vi "niRFUtil MT Resample.vi"(0 "Waveform In":T1={"x0"=0.0, "dx"=1.0, "y"=[]} caption="input complex waveform" {"y" format="%.2f"; "dx" format="%^.2e"; "x0" format="%^.2e"}, 1 "initial sample offset (sec)":dbl format="%.2f", 7 "desired sample rate (Hz)":dbl=1.0 format="%.2f", 11 "error in (no error)":errorcluster, 12 "allowable sample rate error (ppm)":dbl=1.0 format="%.2g", 13 "reset? (T)":bool=TRUE, 14 "flush buffers? (F)":bool) -> (4 "Waveform Out":T1 caption="output complex waveform" {"y" format="%.2f"; "dx" format="%^.2e"; "x0" format="%^.2e"}, 15 "error out":errorcluster)   [LabVIEW 2015, in "niRFUtil.lvlib"]
doc: "Specifies a complex-valued waveform and resamples and/or realigns it based on the input parameters that you specify."
uses:
  niRFUtil.lvlib
  Includes/niRFUtil INC Complex Waveform.ctl
  Includes/niRFUtil INC Complex Array.ctl
  Utilities/niRFUtil MT UTIL Integer Rate Interpolation (Complex SGL).vi
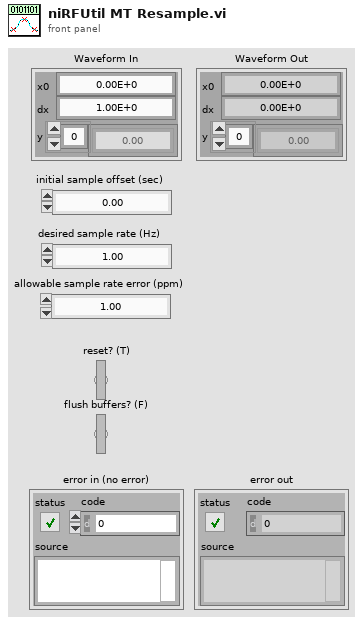
[diagram p1: front panel]
types:
  T1 = typedef "niRFUtil.lvlib/niRFUtil INC Complex Waveform.ctl" = cluster{"x0":dbl, "dx":dbl, "y":T2}
  T2 = typedef "niRFUtil.lvlib/niRFUtil INC Complex Array.ctl" = csg[]
  T3 = enum16{"interpolate", "2-stage interpolate", "decimate", "2-stage decimate", "integer interpolate", "integer decimate", "no resampling"}
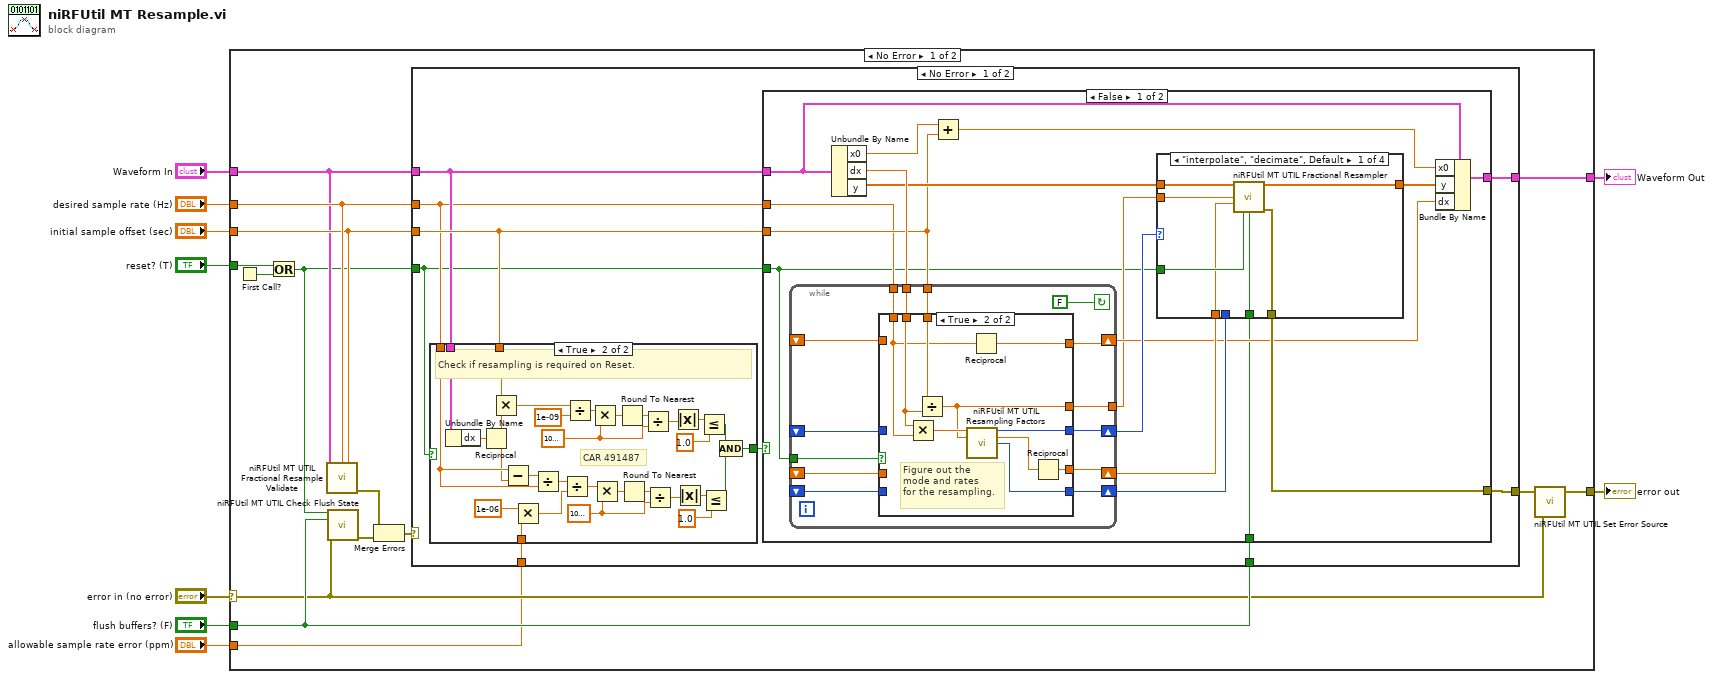
[diagram p0: block diagram]
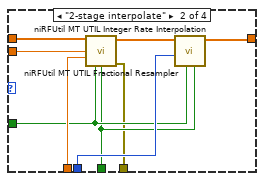
[diagram p3: hidden frame]
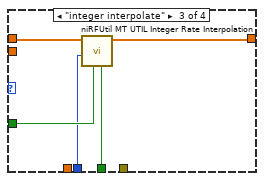
[diagram p4: hidden frame]
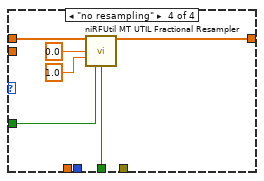
[diagram p5: hidden frame]
diagram:
  n1 = case shown="No Error" "error in (no error)" {
    selector: "error in (no error)" -> [w17 w137]
    tunnel: "desired sample rate (Hz)" -> [w24 _]
    tunnel: "initial sample offset (sec)" -> [w23 _]
    tunnel: "Waveform In" -> [w22 _]
    tunnel: [w19 w137] -> w5
    tunnel: [w21 _] -> w3
    tunnel: "reset? (T)" -> [w12 _]
    tunnel: "flush buffers? (F)" -> [w18 _]
    tunnel: "allowable sample rate error (ppm)" -> [w10 _]
    frame No Error {
      n2 = First Call?() -> (First Call?: T/F=w13:bool)
      n3 = Or(x=w12, y=w13) -> (x .or. y?=w11:bool)
      n4 = call "niRFUtil MT UTIL Fractional Resample Validate.vi"("Waveform In"=w22, "Desired Sample Rate, Hz"=w24, "Sample Phase Offset, sec"=w23) -> ("error out"=w16:errorcluster)  [unwired: 12 out]
      n5 = call "niRFUtil MT UTIL Check Flush State.vi"("reset?"=w11, "flush buffers? (F)"=w18, "error in (no error)"=w17) -> ("error out"=w15:errorcluster)  [unwired: 12 out]
      n6 = Merge Errors(w16, w15) -> (w14:errorcluster)
      n7 = case shown="No Error" w14 {
        selector: w14 -> [_ w136]
        tunnel: w24 -> [w27 _]
        tunnel: w23 -> [w30 _]
        tunnel: w22 -> [w29 _]
        tunnel: [w33 w136] -> w20
        tunnel: [w32 _] -> w21
        tunnel: w11 -> [w25 _]
        tunnel: w18 -> [w31 _]
        tunnel: w10 -> [w28 _]
        frame No Error {
          n8 = case shown="True" w25 {
            tunnel: w30 -> [_ w35]
            tunnel: w29 -> [_ w62]
            tunnel: w28 -> [_ w59]
            tunnel: w27 -> [_ w57]
            tunnel: [_ w56] -> w26
            frame False {
            }
            frame True {
              w44 = 1000000.0 ("y")
              w47 = 1000000.0 ("y")
              # "CAR 491487"
              # "Check if resampling is required on Reset."
              n9 = Unbundle By Name(w62) -> ("dx"=w61:dbl)
              n10 = Reciprocal(x=w61) -> (1/x=w36:dbl)
              n11 = Multiply(x=w35, y=w36) -> (x*y=w34:dbl)
              n12 = Subtract(x=w57, y=w36) -> (x-y=w60:dbl)
              n13 = Multiply(x=1e-06, y=w59) -> (x*y=w51:dbl)
              n14 = Divide(x=w60, y=w57) -> (x/y=w52:dbl)
              n15 = Divide(x=w52, y=w51) -> (x/y=w50:dbl)
              n16 = Divide(x=w34, y=1e-09 ("upper limit")) -> (x/y=w39:dbl)
              n17 = Multiply(x=w39, y=w44) -> (x*y=w42:dbl)
              n18 = Multiply(x=w50, y=w47) -> (x*y=w49:dbl)
              n19 = Round To Nearest(number=w42) -> (nearest integer value=w43:dbl)
              n20 = Round To Nearest(number=w49) -> (nearest integer value=w48:dbl)
              n21 = Divide(x=w43, y=w44) -> (x/y=w45:dbl)
              n22 = Divide(x=w48, y=w47) -> (x/y=w46:dbl)
              n23 = Absolute Value(x=w45) -> (abs(x)=w40:dbl)
              n24 = Absolute Value(x=w46) -> (abs(x)=w54:dbl)
              n25 = Less Or Equal?(x=w40, y=1.0) -> (x <= y?=w38:bool)
              n26 = Less Or Equal?(x=w54, y=1.0) -> (x <= y?=w55:bool)
              n27 = Compound Arithmetic op=AND(w38, w55) -> (w56:bool)
            }
          }
          n28 = case shown="False" w26 {
            tunnel: [w79 _] -> w33
            tunnel: [w75 w135] -> w32
            tunnel: w31 -> [w68 _]
            tunnel: w30 -> [w66 _]
            tunnel: w29 -> [w65 w135]
            tunnel: w27 -> [w64 _]
            tunnel: w25 -> [w63 _]
            frame False {
              n29 = Unbundle By Name(w65) -> ("x0"=w73:dbl, "dx"=w78:dbl, "y"=w71:T2)
              n30 = while {
                tunnel: w64 -> [w119]
                tunnel: w78 -> [w118]
                shift-right: [w117] -> w77
                shift-left: _ -> [w116]
                tunnel: w66 -> [w115]
                shift-right: [w110] -> w69
                shift-left: _ -> [w111]
                shift-right: [w114] -> w76
                shift-left: _ -> [w113]
                shift-right: [w109] -> w70
                shift-left: _ -> [w112]
                tunnel: w63 -> [w108]
                tunnel: [w107] -> w67
                stop <- FALSE continue-if-true
                n31 = case shown="True" w108 {
                  tunnel: w119 -> [_ w128]
                  tunnel: w118 -> [_ w130]
                  tunnel: [w124 w131] -> w117
                  tunnel: w116 -> [w124 _]
                  tunnel: w115 -> [_ w134]
                  tunnel: w111 -> [w122 _]
                  tunnel: [w123 w125] -> w114
                  tunnel: w113 -> [w123 _]
                  tunnel: w112 -> [w121 _]
                  tunnel: [w122 w129] -> w110
                  tunnel: [w121 w127] -> w109
                  tunnel: [_ w126] -> w107
                  frame False {
                  }
                  frame True {
                    # "Figure out the \nmode and rates \nfor the resampling."
                    n32 = Multiply(x=w130, y=w128) -> (x*y=w133:dbl)
                    n33 = Divide(x=w134, y=w130) -> (x/y=w126:dbl)
                    n34 = call "niRFUtil MT UTIL Resampling Factors.vi"("resampling factor"=w133, "initial sample offset"=w126) -> ("resampling mode"=w127:T3, "fractional factor"=w132:dbl, "integer factor"=w131:i32)  [unwired: 1 in, 10 out]
                    n35 = Reciprocal(x=w128) -> (1/x=w129:dbl)
                    n36 = Reciprocal(x=w132) -> (1/x=w125:dbl)
                  }
                }
              }
              n37 = Add(x=w73, y=w66) -> (x+y=w72:dbl)
              n38 = case shown="\"interpolate\", \"decimate\", Default" w70 {
                tunnel: [w85 w91 w99 w105] -> w74
                tunnel: w71 -> [w86 w95 w100 w106]
                tunnel: [w80 w87 _ _] -> w79
                tunnel: w77 -> [_ w90 w96 _]
                tunnel: w76 -> [w81 w93 _ _]
                tunnel: w63 -> [w84 w89 w98 w102]
                tunnel: w68 -> [w83 w88 w97 w101]
                tunnel: w67 -> [w82 w94 _ _]
                frame "interpolate", "decimate", Default {
                  n39 = call "niRFUtil MT UTIL Fractional Resampler.vi"("samples in"=w86, "offset"=w82, "rate factor"=w81, "reset"=w84, "flush"=w83) -> ("samples out"=w85:T2, "error out"=w80:errorcluster)  [unwired: 8 in, 1 out]
                }
                frame "2-stage interpolate" {
                  n40 = call "niRFUtil MT UTIL Fractional Resampler.vi"("samples in"=w95, "offset"=w94, "rate factor"=w93, "reset"=w89, "flush"=w88) -> ("samples out"=w92:T2, "error out"=w87:errorcluster)  [unwired: 8 in, 1 out]
                  n41 = call-poly "niRFUtil MT UTIL Integer Rate Interpolation.vi"("flush buffers? (F)"=w88, "reset? (T)"=w89, "interpolation factor"=w90, "input[]"=w92) -> ("output[]"=w91:csg[])  [unwired: 6 in, 1 out]
                }
                frame "integer interpolate" {
                  n42 = call-poly "niRFUtil MT UTIL Integer Rate Interpolation.vi"("flush buffers? (F)"=w97, "reset? (T)"=w98, "interpolation factor"=w96, "input[]"=w100) -> ("output[]"=w99:csg[])  [unwired: 6 in, 1 out]
                }
                frame "no resampling" {
                  n43 = call "niRFUtil MT UTIL Fractional Resampler.vi"("samples in"=w106, "offset"=0.0, "rate factor"=1.0, "reset"=w102, "flush"=w101) -> ("samples out"=w105:T2)  [unwired: 8 in, 2 out]
                }
              }
              n44 = Bundle By Name(cluster=w65, "x0"=w72, "y"=w74, "dx"=w69) -> (w75:T1)
            }
            frame True {
            }
          }
        }
        frame Error {
        }
      }
      n45 = call "niRFUtil MT UTIL Set Error Source.vi"("initial error in (no error)"=w17, "final error in (no error)"=w20) -> ("error out"=w19:errorcluster)  [unwired: 3 out]
    }
    frame Error {
    }
  }
  "error out" <- w5
  "Waveform Out" <- w3
